vi "testTime.vi"() -> ()   [LabVIEW 2014]
panel:
  in  "stop":bool
  out "date/time string":string
  in  "Action":enum16{"Count", "Stop", "Reset"}(ring)
  in  "start":bool
  in  "reset":bool
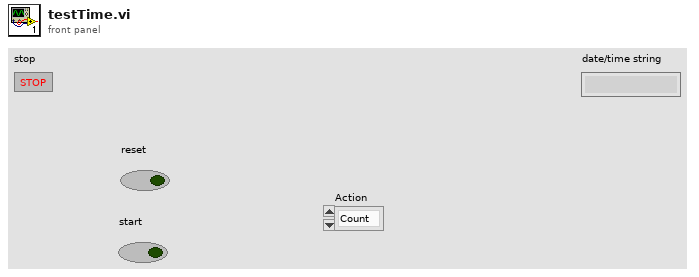
[diagram p1: front panel]
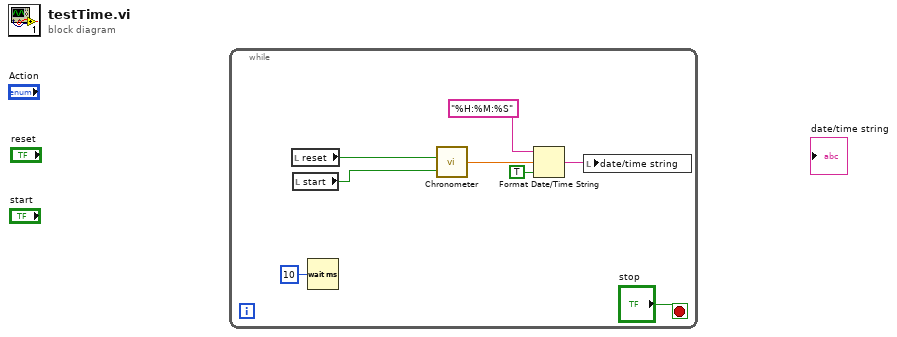
[diagram p0: block diagram]
diagram:
  n1 = while {
    stop <- "stop" stop-if-true
    n2 = local read "reset"() -> (w2:bool)
    n3 = local read "start"() -> (w1:bool)
    n4 = Wait (ms)(milliseconds to wait=u32 10) -> ()  [unwired: 1 out]
    n5 = call "Chronometer.vi"("start"=w1, "reset"=w2) -> ("Time"=w7:dbl)
    n6 = Format Date/Time String(time format string (%c)="%H:%M:%S", seconds (now)=w7, UTC format=TRUE) -> (date/time string=w5:string)
    n7 = local write "date/time string"(w5) -> ()
  }
